vi "Slot1Dialog.vi"(8 "Error In":errorcluster, 11 "Slot 1 Configuration In":T1) -> (0 "Error Out":errorcluster, 2 "Cancelled?":bool, 3 "Slot 1 Configuration Out":T1)   [LabVIEW 2012]
uses:
  SlotConfiguration.ctl
  BankConfiguration.ctl
  libs/LV-Utilities/LV-Utilities.lvlib
panel:
  in  "CANCEL":bool
  in  "DONE":bool
  in  "Bank D Channel Names":string[](array[string])
  in  "Bank D Name":string="Bank D"
  in  "Bank C Channel Names":string[](array[string])
  in  "Bank C Name":string="Bank C"
  in  "Bank B Channel Names":string[](array[string])
  in  "Bank B Name":string="Bank B"
  in  "Bank A Channel Names":string[](array[string])
  in  "Bank A Name":string="Bank A"
  # "SLOT 1"
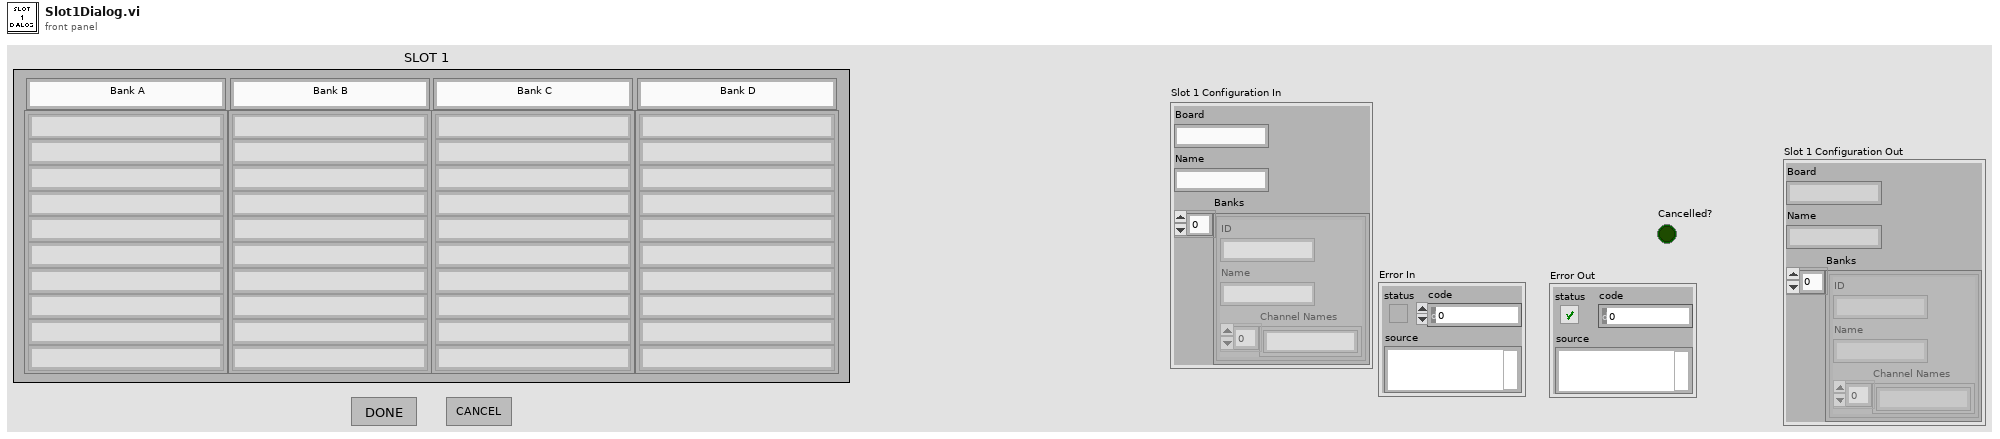
[diagram p1: front panel]
types:
  T1 = typedef "SlotConfiguration.ctl" = cluster{"Board":string, "Name":string, "Banks":T2[]}
  T2 = typedef "BankConfiguration.ctl" = cluster{"ID":string, "Name":string, "Channel Names":string[]}
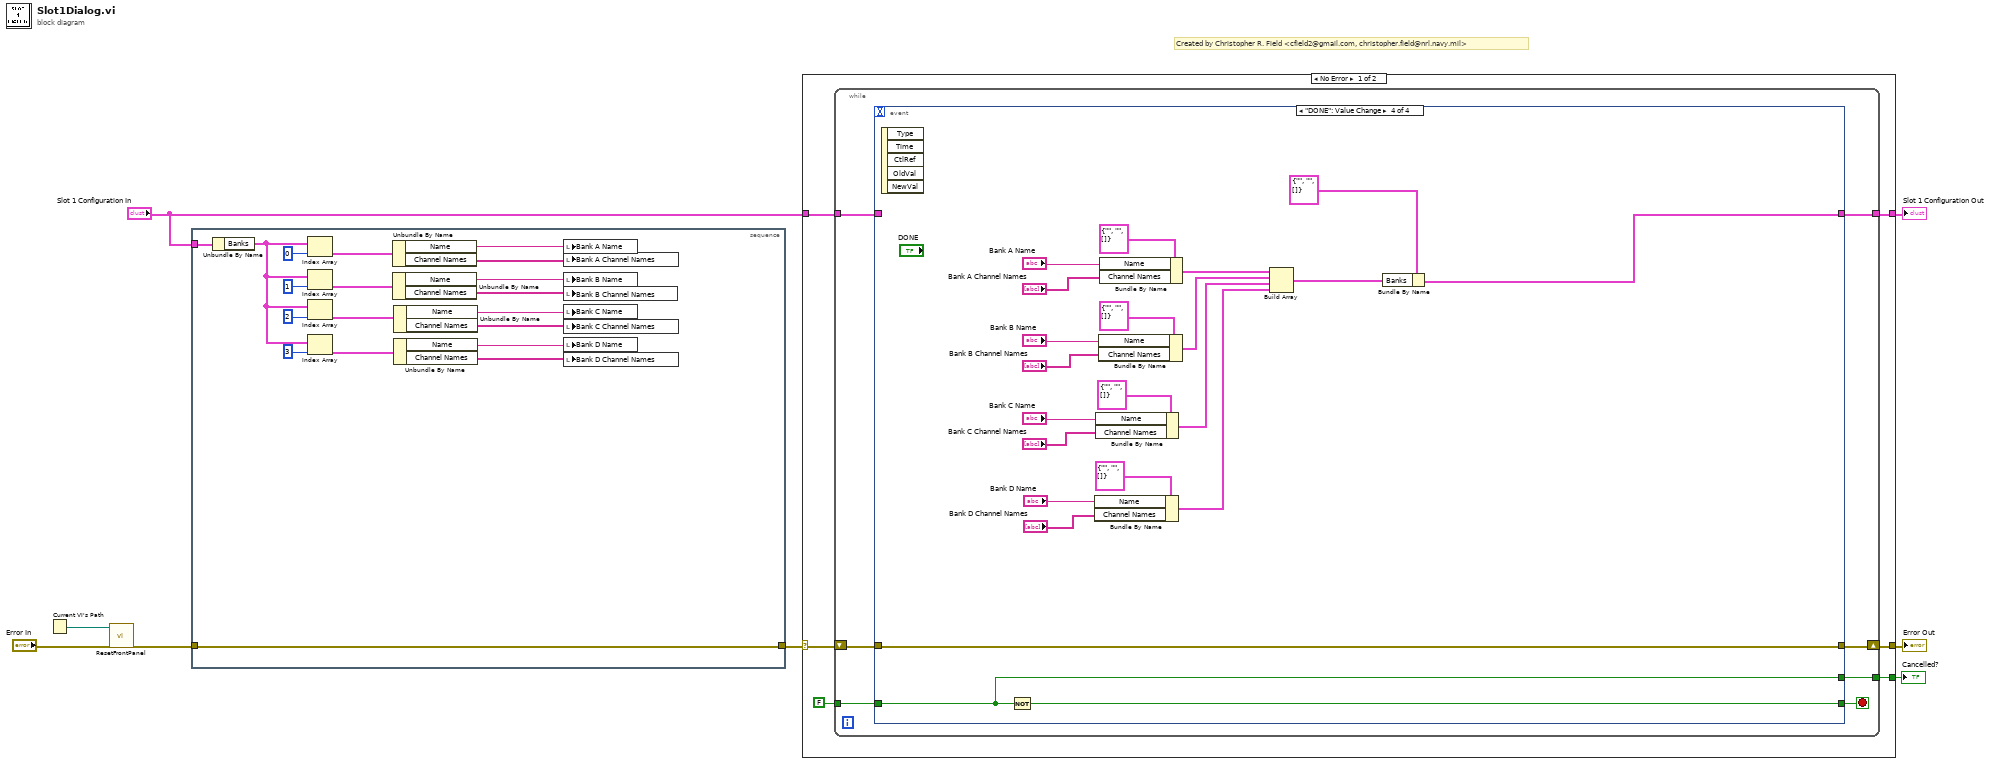
[diagram p0: block diagram]
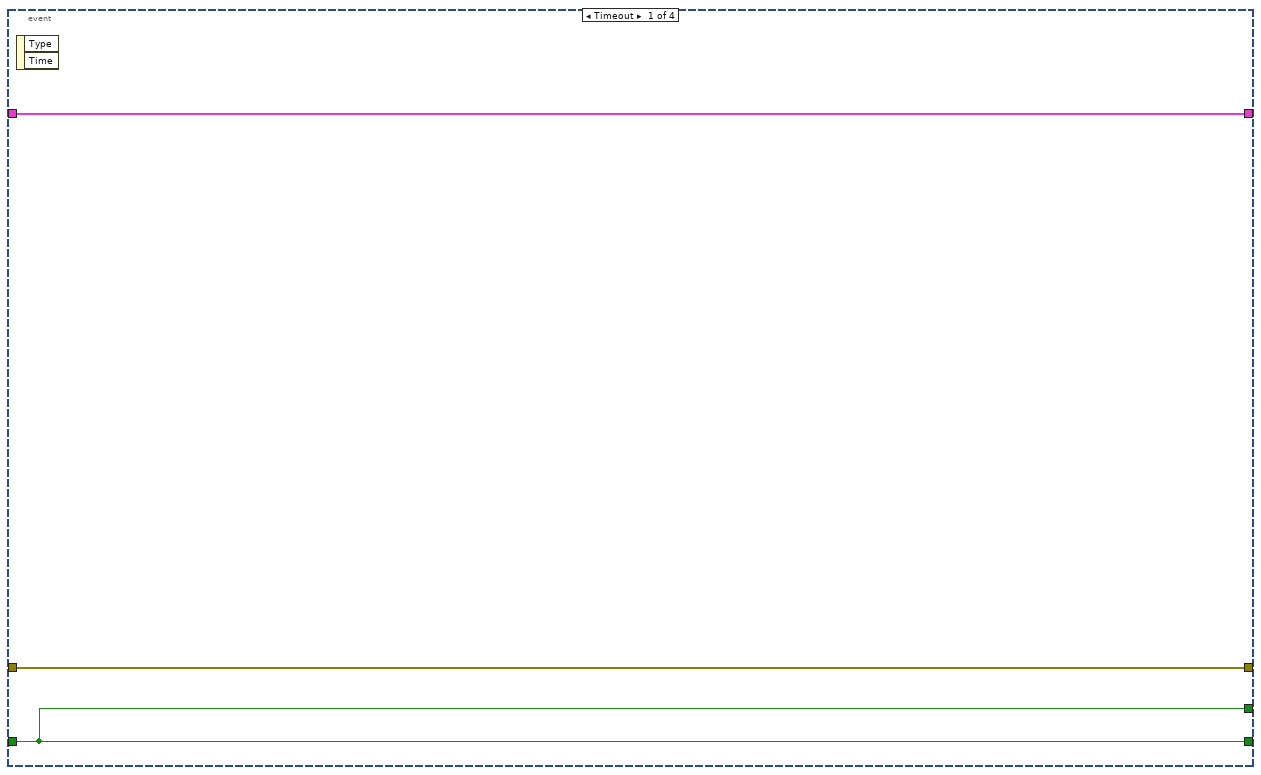
[diagram p2: hidden frame]
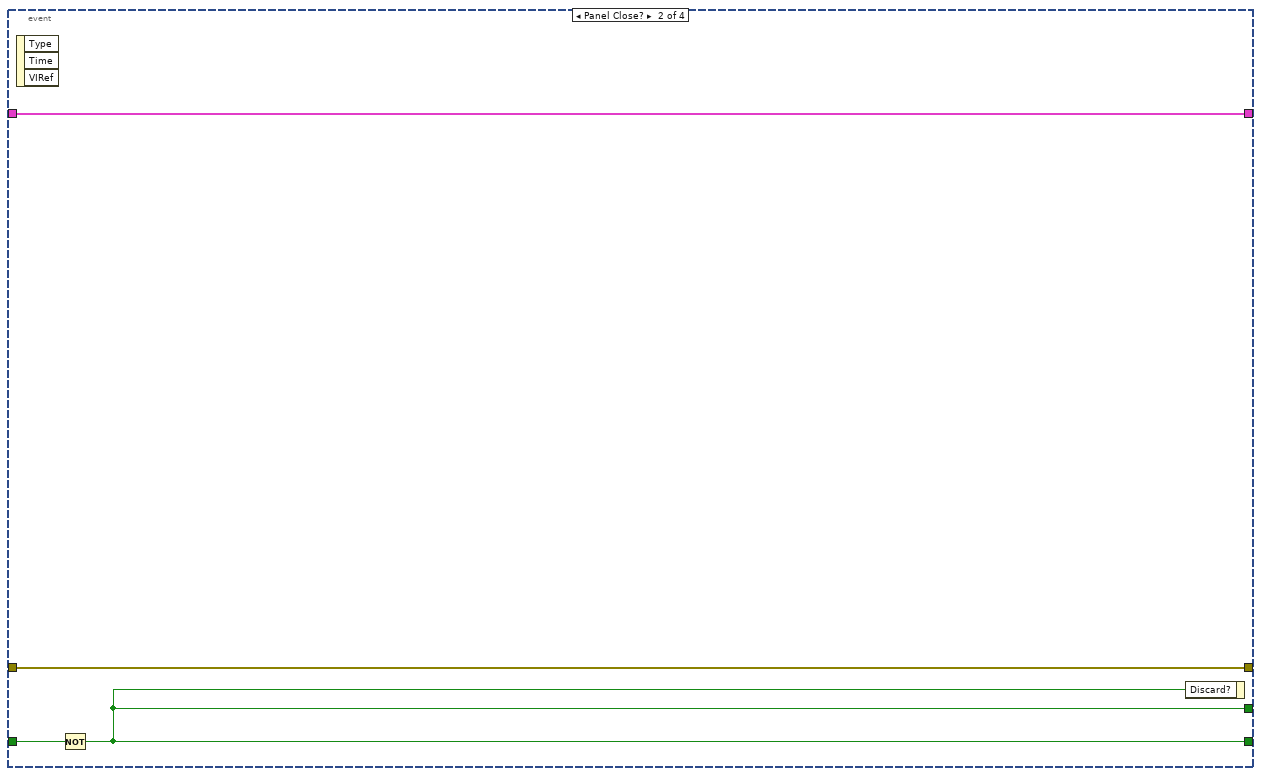
[diagram p3: hidden frame]
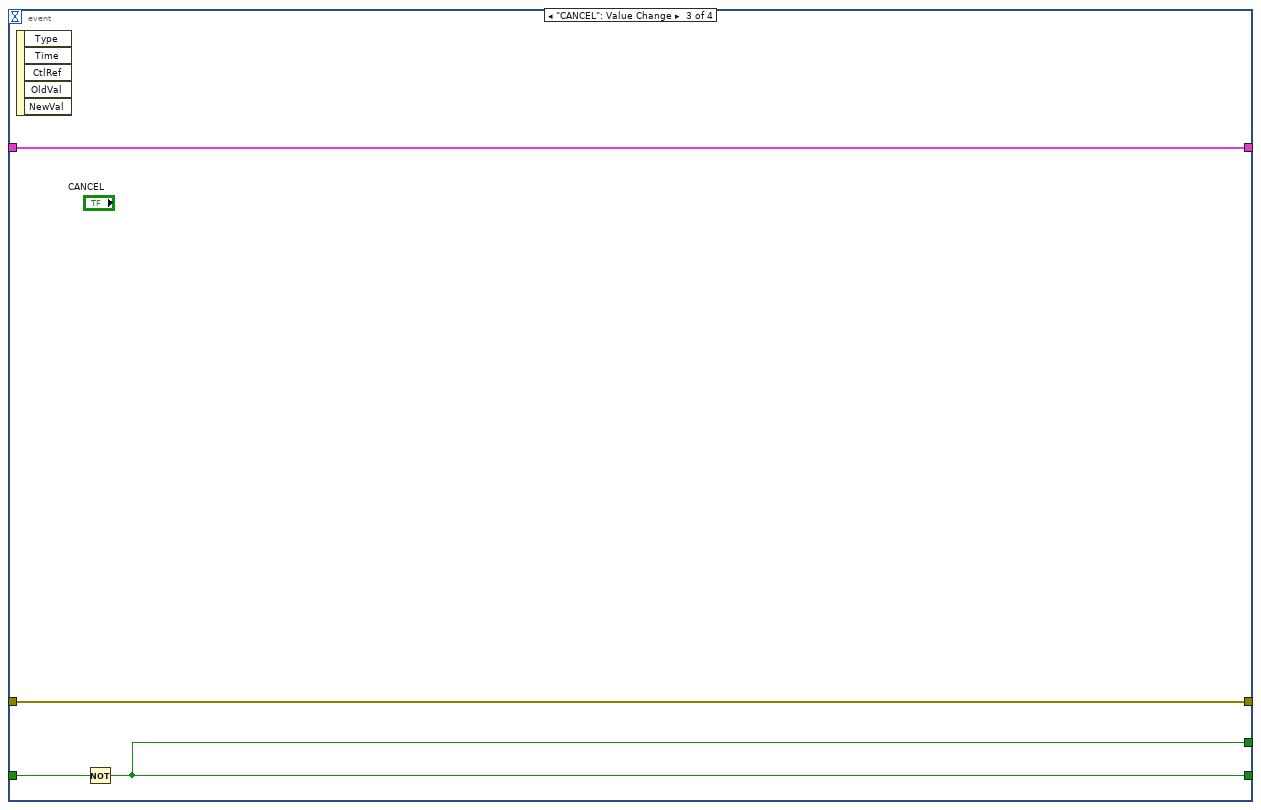
[diagram p4: hidden frame]
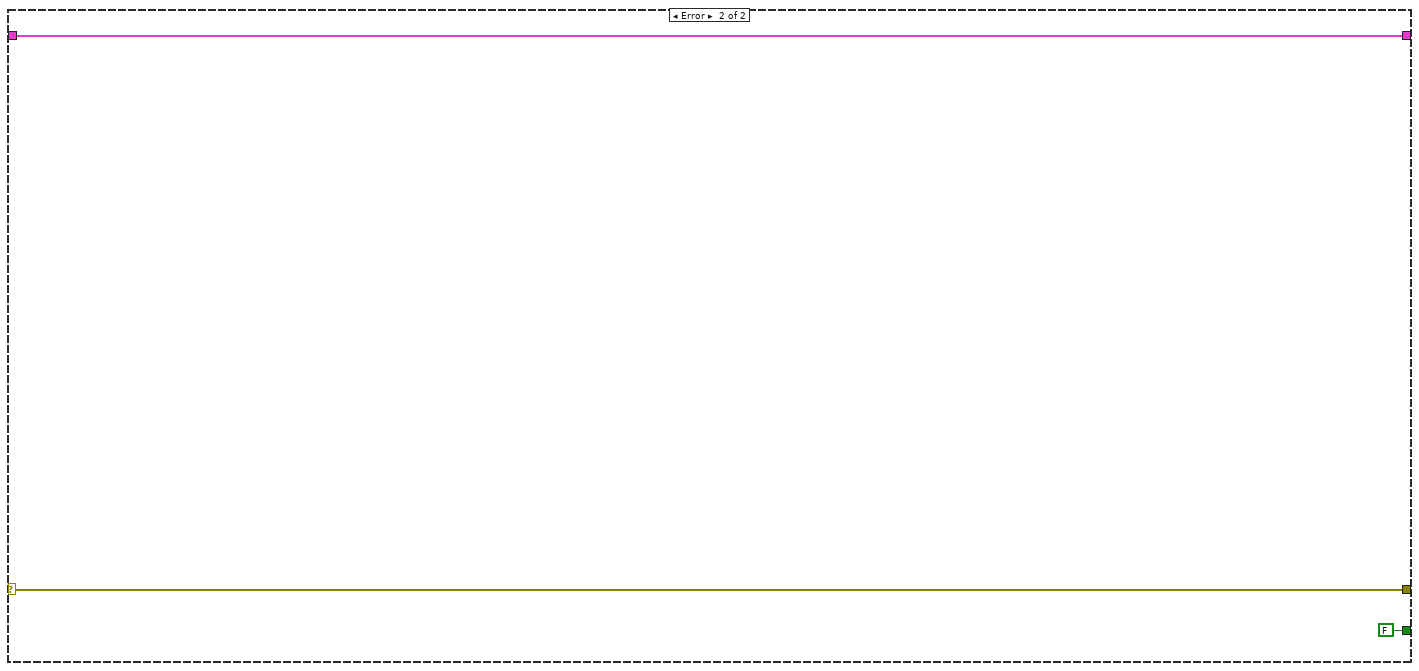
[diagram p5: hidden frame]
diagram:
  # "Created by Christopher R. Field <cfield2@gmail.com, christopher.field@nrl.navy.mil>"
  n1 = Current VI's Path() -> (path=w5:path)
  n2 = call "ResetFrontPanel.vi"("Error In"="Error In", "VI Path"=w5) -> ("Error Out"=w8:errorcluster)  [unwired: 9 in]
  n3 = stacked-sequence {
    tunnel: w8 -> [w27]
    tunnel: [w27] -> w7
    tunnel: "Slot 1 Configuration In" -> [w26]
    frame #0 {
      n4 = Unbundle By Name(w26) -> ("Banks"=w20:T2[])
      n5 = Index Array(array=w20, index=0) -> (element=w24:T2)
      n6 = Index Array(array=w20, index=1) -> (element=w19:T2)
      n7 = Index Array(array=w20, index=2) -> (element=w18:T2)
      n8 = Index Array(array=w20, index=3) -> (element=w17:T2)
      n9 = Unbundle By Name(w24) -> ("Name"=w16:string, "Channel Names"=w15:string[])
      n10 = Unbundle By Name(w19) -> ("Name"=w14:string, "Channel Names"=w13:string[])
      n11 = Unbundle By Name(w18) -> ("Name"=w12:string, "Channel Names"=w11:string[])
      n12 = Unbundle By Name(w17) -> ("Name"=w10:string, "Channel Names"=w9:string[])
      n13 = local write "Bank A Name"(w16) -> ()
      n14 = local write "Bank A Channel Names"(w15) -> ()
      n15 = local write "Bank B Name"(w14) -> ()
      n16 = local write "Bank B Channel Names"(w13) -> ()
      n17 = local write "Bank C Name"(w12) -> ()
      n18 = local write "Bank C Channel Names"(w11) -> ()
      n19 = local write "Bank D Name"(w10) -> ()
      n20 = local write "Bank D Channel Names"(w9) -> ()
    }
  }
  n21 = case shown="No Error" w7 {
    selector: w7 -> [w32 w76]
    tunnel: [w31 w76] -> w4
    tunnel: [w30 FALSE] -> w3
    tunnel: "Slot 1 Configuration In" -> [w29 w74]
    tunnel: [w28 w74] -> w1
    frame No Error {
      n22 = while {
        tunnel: FALSE -> [w40]
        shift-right: [w37] -> w31
        shift-left: w32 -> [w38]
        tunnel: [w36] -> w30
        tunnel: w29 -> [w35]
        tunnel: [w34] -> w28
        stop <- w39 stop-if-true
        n23 = event shown="[3] \"DONE\": Value Change" {
          selector: _ -> [_ _ _ _]
          dyn-events: _ -> [_ _ _ _]
          timeout: _ -> [_ _ _ _]
          tunnel: w40 -> [w42 w46 w50 w71]
          tunnel: [w42 w45 w49 w72] -> w39
          tunnel: w38 -> [w43 w47 w51 w73]
          tunnel: [w43 w47 w51 w73] -> w37
          tunnel: [w42 w45 w49 w71] -> w36
          tunnel: w35 -> [w41 w44 w48 _]
          tunnel: [w41 w44 w48 w57] -> w34
          event Timeout {
            n24 = event-data() -> ()  [unwired: 1 in, 2 out]
          }
          event Panel Close? {
            n25 = event-data() -> ()  [unwired: 1 in, 3 out]
            n26 = Not(x=w46) -> (.not. x?=w45:bool)
            n27 = event-data("Discard?"=w45) -> ()  [unwired: 1 in, 1 out]
          }
          event "CANCEL": Value Change {
            n28 = event-data() -> ()  [unwired: 1 in, 5 out]
            n29 = Not(x=w50) -> (.not. x?=w49:bool)
          }
          event "DONE": Value Change {
            n30 = event-data() -> ()  [unwired: 1 in, 5 out]
            n31 = Not(x=w71) -> (.not. x?=w72:bool)
            n32 = Bundle By Name(cluster=T2 {"ID"="", "Name"="", "Channel Names"=[]} ("Bank Configuration"), "Name"="Bank D Name", "Channel Names"="Bank D Channel Names") -> (w53:T2)
            n33 = Bundle By Name(cluster=T2 {"ID"="", "Name"="", "Channel Names"=[]} ("Bank Configuration"), "Name"="Bank C Name", "Channel Names"="Bank C Channel Names") -> (w54:T2)
            n34 = Bundle By Name(cluster=T2 {"ID"="", "Name"="", "Channel Names"=[]} ("Bank Configuration"), "Name"="Bank B Name", "Channel Names"="Bank B Channel Names") -> (w55:T2)
            n35 = Bundle By Name(cluster=T2 {"ID"="", "Name"="", "Channel Names"=[]} ("Bank Configuration"), "Name"="Bank A Name", "Channel Names"="Bank A Channel Names") -> (w56:T2)
            n36 = Build Array(w56, w55, w54, w53) -> (w52:T2[])
            n37 = Bundle By Name(cluster=T1 {"Board"="", "Name"="", "Banks"=[]} ("Slot 1 Configuration"), "Banks"=w52) -> (w57:T1)
          }
        }
      }
    }
    frame Error {
    }
  }
  "Error Out" <- w4
  "Cancelled?" <- w3
  "Slot 1 Configuration Out" <- w1
